vi "Mask Actions.vi"(6 "Auto Align":T1 {"Alignment Type (8: None)" items=["EYEAMI", "EYECMI", "EYENRZ", "FANWidth", "FAPeriod", "FAPWidth", "FYNWidth", "FYPWidth", "None", "NWidth", "PWidth", "TMax", "TMin"]}, 8 "error in (no error)":errorcluster, 9 "Filename":string, 10 "Actions (0: Align)":i32(ring) items=["Align", "Create AutoMask", "Save AutoMask", "Load Mask", "Delete Mask", "Invert Mask", "Revert Mask"], 11 "VISA resource name":refnum<visa-resource-name>) -> (0 "error out":errorcluster, 3 "VISA resource name out":refnum<visa-resource-name>)   [LabVIEW 2009, in "Agilent 8000 Series.lvlib"]
doc: "Performs various mask and Automask actions."
uses:
  Agilent 8000 Series.lvlib
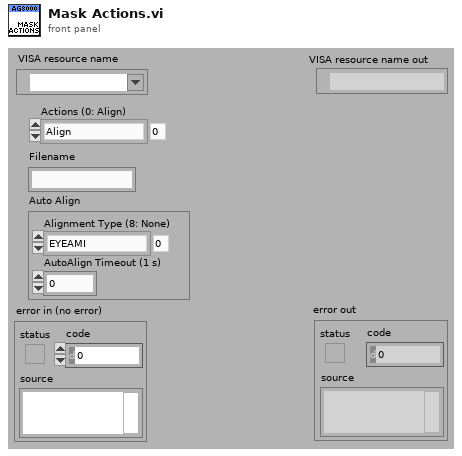
[diagram p1: front panel]
types:
  T1 = cluster{"Alignment Type (8: None)":i32, "AutoAlign Timeout (1 s)":dbl}
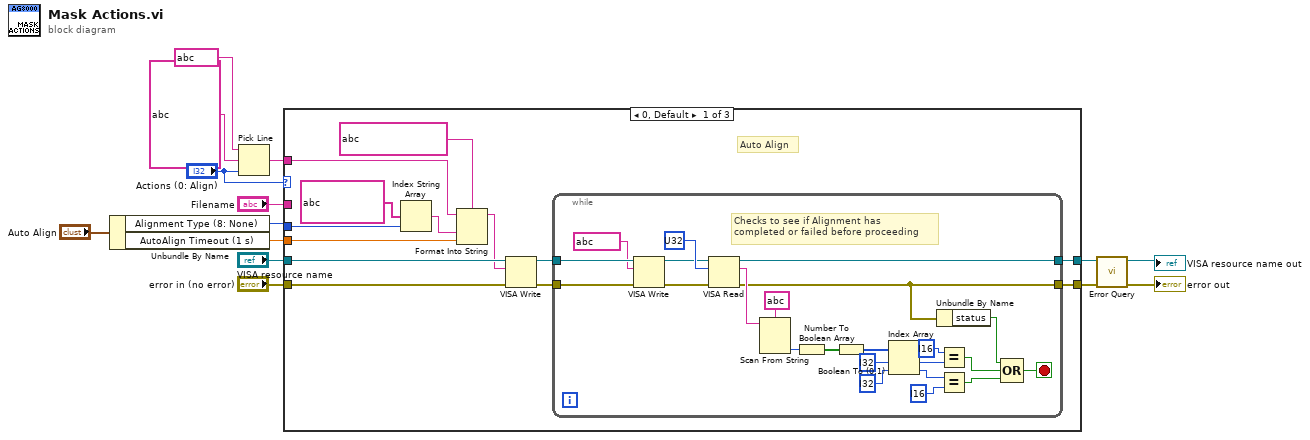
[diagram p0: block diagram]
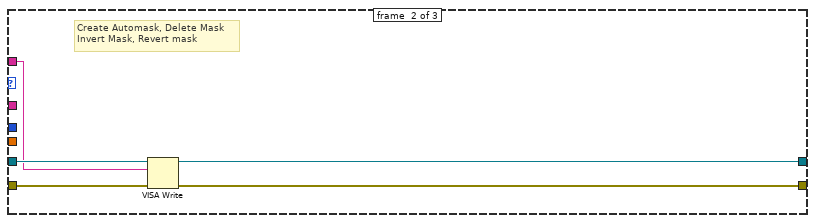
[diagram p2: hidden frame]
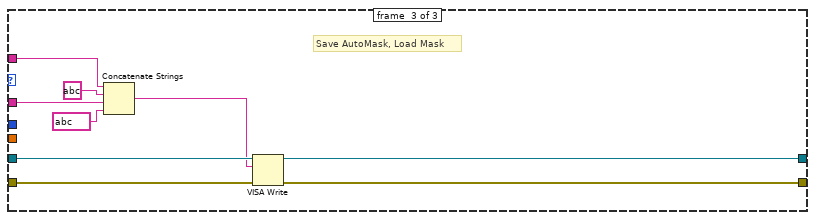
[diagram p3: hidden frame]
diagram:
  n1 = Unbundle By Name("Auto Align") -> ("Alignment Type (8: None)"=w9:i32, "AutoAlign Timeout (1 s)"=w8:dbl)
  n2 = Pick Line(string ("")=string ?, multi-line string=string ?, line index="Actions (0: Align)") -> (output string=w7:string)
  n3 = case shown="0, Default" "Actions (0: Align)" {
    tunnel: "Filename" -> [_ _ w64]
    tunnel: w9 -> [w24 _ _]
    tunnel: w8 -> [w23 _ _]
    tunnel: w7 -> [w22 w53 w61]
    tunnel: "VISA resource name" -> [w21 w55 w60]
    tunnel: "error in (no error)" -> [w20 w54 w59]
    tunnel: [w16 w52 w58] -> w4
    tunnel: [w15 w51 w57] -> w3
    frame #0 {
      # "Auto Align"
      n4 = Index String Array(1:w24, 2:string[] ? ("string array")) -> (0:w25:string)  [unwired: 1 in]
      n5 = Format Into String(format string=string ?, initial string=w22, w25, w23) -> (resulting string=w19:string)  [unwired: 1 in, 1 out]
      n6 = VISA Write(VISA resource name=w21, write buffer=w19, error in (no error)=w20) -> (VISA resource name out=w18:refnum<visa-resource-name>, error out=w17:errorcluster)  [unwired: 1 out]
      n7 = while {
        tunnel: w18 -> [w32]
        tunnel: w17 -> [w31]
        tunnel: [w43] -> w16
        tunnel: [w36] -> w15
        stop <- w37 stop-if-true
        # "Checks to see if Alignment has\ncompleted or failed before proceeding"
        n8 = VISA Write(VISA resource name=w32, write buffer=string ?, error in (no error)=w31) -> (VISA resource name out=w30:refnum<visa-resource-name>, error out=w29:errorcluster)  [unwired: 1 out]
        n9 = VISA Read(VISA resource name=w30, byte count=u32 ?, error in (no error)=w29) -> (VISA resource name out=w43:refnum<visa-resource-name>, read buffer=w49:string, error out=w36:errorcluster)  [unwired: 1 out]
        n10 = Scan From String(format string=string ?, input string=w49) -> (output 1=w46:i32)  [unwired: 3 in, 3 out]
        n11 = Number To Boolean Array(number=w46) -> (Boolean array=w47:bool[])
        n12 = Boolean To (0,1)(Boolean=w47) -> (0, 1=w45:i16[])
        n13 = Index Array(array=w45, index #1=i32 ? ("index"), index #2=i32 ? ("index")) -> (element #1=w41:i16, element #2=w39:i16)
        n14 = Unbundle By Name(w36) -> ("status"=w33:bool)
        n15 = Equal?(x=i16 ? ("y"), y=w41) -> (x = y?=w34:bool)
        n16 = Equal?(x=w39, y=i16 ?) -> (x = y?=w35:bool)
        n17 = Compound Arithmetic op=OR(w33, w34, w35) -> (w37:bool)
      }
    }
    frame #1 {
      # "Create Automask, Delete Mask\nInvert Mask, Revert mask"
      n18 = VISA Write(VISA resource name=w55, write buffer=w53, error in (no error)=w54) -> (VISA resource name out=w52:refnum<visa-resource-name>, error out=w51:errorcluster)  [unwired: 1 out]
    }
    frame #2 {
      # "Save AutoMask, Load Mask"
      n19 = Concatenate Strings(w61, string ? ("string"), w64, string ? ("string")) -> (w56:string)
      n20 = VISA Write(VISA resource name=w60, write buffer=w56, error in (no error)=w59) -> (VISA resource name out=w58:refnum<visa-resource-name>, error out=w57:errorcluster)  [unwired: 1 out]
    }
  }
  n21 = call "Error Query.vi"("error in (no error)"=w3, "VISA resource name"=w4) -> ("error out"=→"error out":errorcluster, "VISA resource name out"=→"VISA resource name out":refnum<visa-resource-name>)  [unwired: 6 in, 2 out]
